vi "String Hex to Interger Hex.vi"(10 "Hex Display Input":string) -> (2 "Integer Decimal Equivalent":i32 format="%.0x")   [LabVIEW 2020]
panel:
  # "This VI converts the hexadecimal representation of a string to its integer decimal equivalent.\n\nSteps to run VI:\n1. Enter a hex value in the control.\n2. Run the VI."
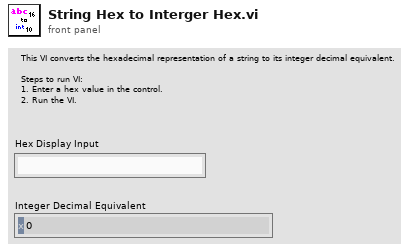
[diagram p1: front panel]
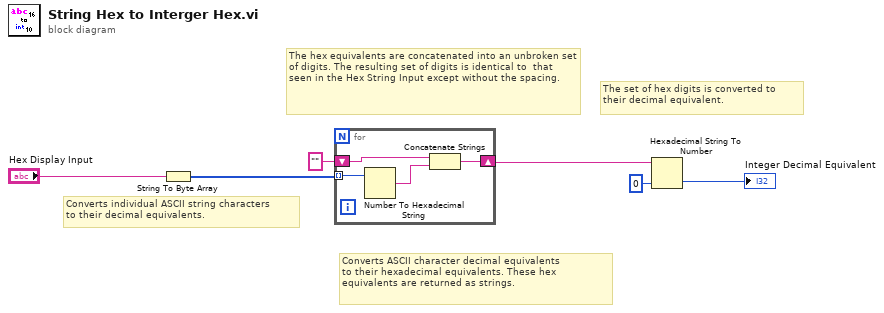
[diagram p0: block diagram]
diagram:
  # "The set of hex digits is converted to their decimal equivalent."
  # "The hex equivalents are concatenated into an unbroken set of digits. The resulting set of digits is identical to  that seen in the Hex String Input except without the spacing."
  # "Converts ASCII character decimal equivalents\nto their hexadecimal equivalents. These hex equivalents are returned as strings."
  # "Converts individual ASCII string characters \nto their decimal equivalents."
  n1 = String To Byte Array(string="Hex Display Input") -> (unsigned byte array=w1:u8[])
  n2 = for {
    tunnel: w1 -> [w10] mode=indexing
    shift-right: [w7] -> w3
    shift-left: "" -> [w8]
    n3 = Number To Hexadecimal String(2:w10) -> (0:w9:string)  [unwired: 1 in]
    n4 = Concatenate Strings(w8, w9) -> (w7:string)
  }
  n5 = Hexadecimal String To Number(string=w3, default (0uL)=0 ("default (0 U32)")) -> (number=→"Integer Decimal Equivalent":i32)  [unwired: 1 in, 1 out]
